vi "Parse-element.vi"(8 "error in (no error)":errorcluster, 10 "String in":string, 11 "Element-XML in":refnum<class "LongDelay.lvclass">) -> (0 "error out":errorcluster, 1 "Valid element?":bool, 2 "Remaining string":string, 3 "Element-XML out":refnum<class "LongDelay.lvclass">)   [LabVIEW 2013, in "MaterialCharacterization.lvlib" / "LongDelay.lvclass"]
uses:
  LongDelay.lvclass
  LongDelay.lvclass/LongDelay.ctl
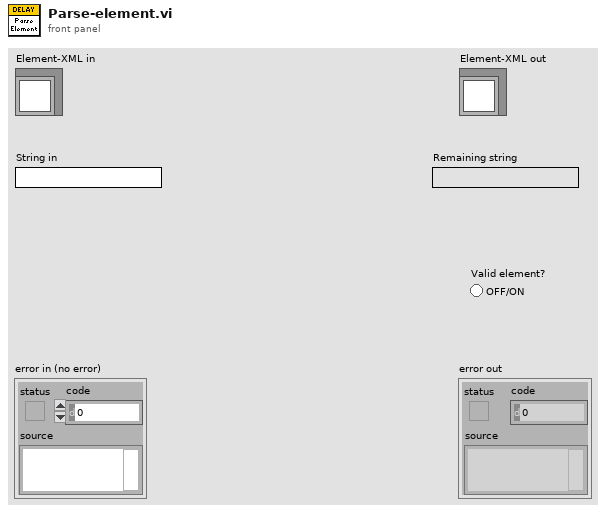
[diagram p1: front panel]
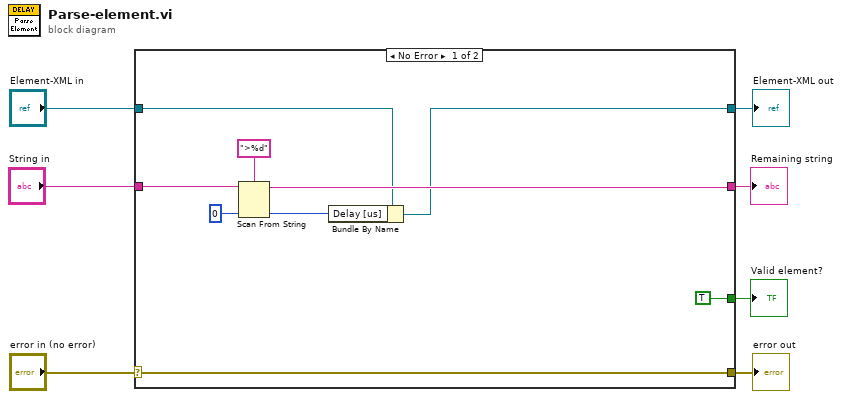
[diagram p0: block diagram]
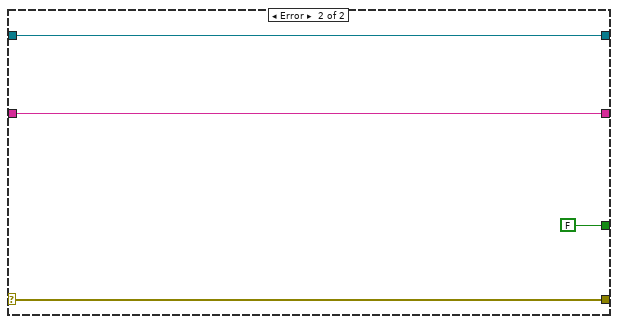
[diagram p2: hidden frame]
diagram:
  n1 = case shown="No Error" "error in (no error)" {
    selector: "error in (no error)" -> [w16 w20]
    tunnel: [w16 w20] -> w6
    tunnel: [w9 w19] -> w4
    tunnel: "Element-XML in" -> [w10 w19]
    tunnel: "String in" -> [w12 w17]
    tunnel: [TRUE FALSE] -> w2
    tunnel: [w11 w17] -> w1
    frame No Error {
      n2 = Scan From String(format string=">%d", input string=w12, default 1=i64 0 ("default value 1")) -> (remaining string=w11:string, output 1=w13:i64)  [unwired: 2 in, 2 out]
      n3 = Bundle By Name(cluster=w10, "Delay [us]"=w13) -> (w9:refnum<class "LongDelay.lvclass">)
    }
    frame Error {
    }
  }
  "error out" <- w6
  "Element-XML out" <- w4
  "Valid element?" <- w2
  "Remaining string" <- w1
